vi "MultiChannel Moving Average Filter PtByPt 2.vi"(10 "sample?":bool, 11 "x":dbl[](array[numeric])) -> (3 "Array":dbl[](array[numeric]))   [LabVIEW 2011, in "Filter VIs.lvlib"]
uses:
  Filter VIs.lvlib
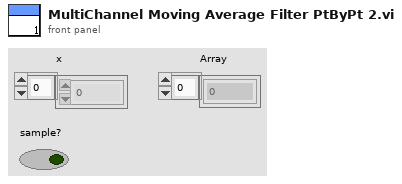
[diagram p1: front panel]
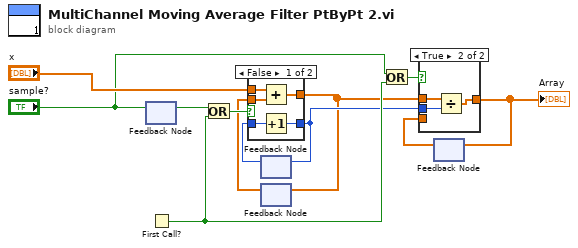
[diagram p0: block diagram]
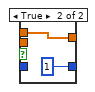
[diagram p3: hidden frame]
diagram:
  n1 = feedback #1() -> (w12:bool)  [unwired: 1 in]
  n2 = feedback-in #1("sample?") -> ()
  n3 = First Call?() -> (First Call?: T/F=w6:bool)
  n4 = Or(x=w12, y=w6) -> (x .or. y?=w11:bool)
  n5 = feedback #2() -> (w8:u64)  [unwired: 1 in]
  n6 = feedback #3() -> (w9:dbl[])  [unwired: 1 in]
  n7 = case shown="False" w11 {
    tunnel: [w17 u64 1 ("n")] -> w2
    tunnel: w8 -> [w16 _]
    tunnel: w9 -> [w15 _]
    tunnel: "x" -> [w14 w18]
    tunnel: [w13 w18] -> w1
    frame False {
      n8 = Add(x=w14, y=w15) -> (x+y=w13:dbl[])
      n9 = Increment(x=w16) -> (x+1=w17:u64)
    }
    frame True {
    }
  }
  n10 = feedback-in #2(w2) -> ()
  n11 = feedback-in #3(w1) -> ()
  n12 = Or(x="sample?", y=w6) -> (x .or. y?=w5:bool)
  n13 = feedback #4() -> (w3:dbl[])  [unwired: 1 in]
  n14 = case shown="True" w5 {
    tunnel: [w20 w23] -> w4
    tunnel: w3 -> [w20 _]
    tunnel: w2 -> [_ w22]
    tunnel: w1 -> [_ w21]
    frame False {
    }
    frame True {
      n15 = Divide(x=w21, y=w22) -> (x/y=w23:dbl[])
    }
  }
  "Array" <- w4
  n16 = feedback-in #4(w4) -> ()
